vi "APS wait trigger sampling.vi"(6 "DataArr":T1, 7 "TimeOutMs":i32, 8 "error in (no error)":errorcluster caption="错误输入（无错误）", 9 "PreTrgLen":i32, 10 "Length":i32, 11 "Board_ID":i32) -> (0 "error out":errorcluster caption="错误输出", 3 "function return":i32, 4 "DataArr out":T1)   [LabVIEW 2011, in "APS168.lvlib"]
doc: "I32 FNTYPE APS_wait_trigger_sampling( I32 Board_ID, I32 Length, I32 PreTrgLen, I32 TimeOutMs, STR_SAMP_DATA_4CH *DataArr );"
uses:
  APS168.lvlib
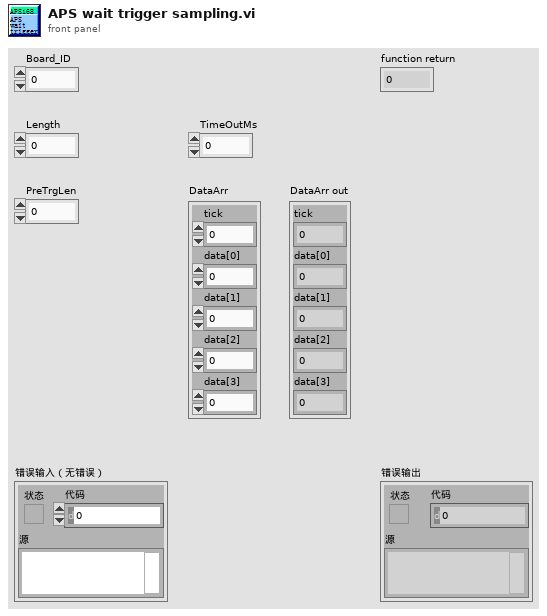
[diagram p1: front panel]
types:
  T1 = cluster{"tick":i32, "data[0]":i32, "data[1]":i32, "data[2]":i32, "data[3]":i32}
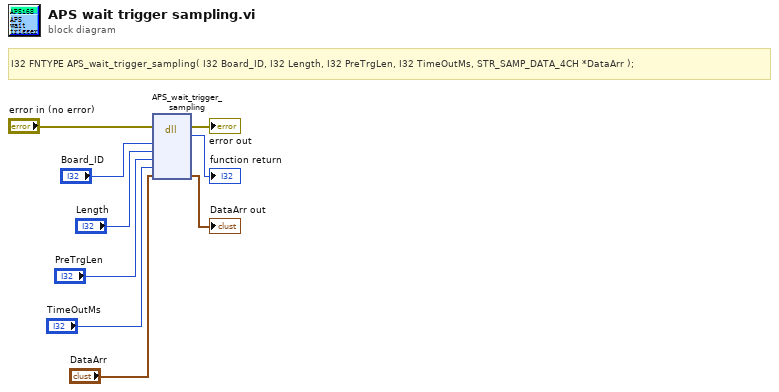
[diagram p0: block diagram]
diagram:
  # "I32 FNTYPE APS_wait_trigger_sampling( I32 Board_ID, I32 Length, I32 PreTrgLen, I32 TimeOutMs, STR_SAMP_DATA_4CH *DataArr );"
  n1 = dll-call lib="PTH1Labs E软件ADLINK 204CAPS_1_7_1_LIB line 连续运动204APS168.*" fn="APS_wait_trigger_sampling"(error in="error in (no error)", "Board_ID"="Board_ID", "Length"="Length", "PreTrgLen"="PreTrgLen", "TimeOutMs"="TimeOutMs", "DataArr"="DataArr") -> (error out=→"error out":errorcluster, →"function return":i32, "DataArr"=→"DataArr out":T1)  [unwired: 6 in, 1 out]
